vi "pwm事件.vi"(8 "error in (no error)":errorcluster caption="错误输入（无错误）", 9 "事件数据":cluster{"frequency":dbl, "duty cycle":dbl}, 10 "枚举":T1) -> (0 "error out":errorcluster, 3 "user event":refnum<user-event>)   [LabVIEW 2012]
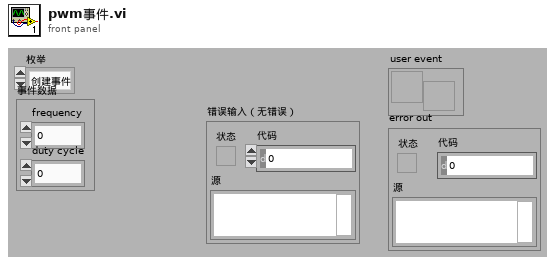
[diagram p1: front panel]
types:
  T1 = typedef "控件 2.ctl" = enum16{"创建事件", "产生事件", "销毁事件"}
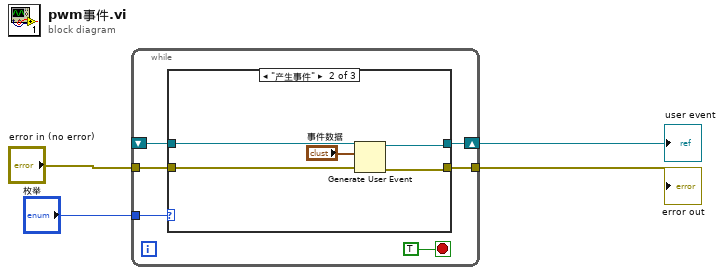
[diagram p0: block diagram]
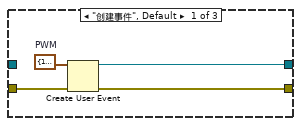
[diagram p2: hidden frame]
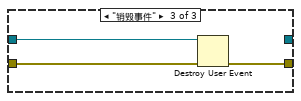
[diagram p3: hidden frame]
diagram:
  n1 = while {
    tunnel: "枚举" -> [w9]
    shift-right: [w8] -> w3
    shift-left: _ -> [w7]
    tunnel: "error in (no error)" -> [w6]
    tunnel: [w5] -> w2
    stop <- TRUE stop-if-true
    n2 = case shown="\"产生事件\"" w9 {
      tunnel: [w14 w17 _] -> w8
      tunnel: w7 -> [_ w19 w22]
      tunnel: w6 -> [w13 w16 w21]
      tunnel: [w12 w15 w20] -> w5
      frame "创建事件", Default {
        w11 = cluster{"frequency":dbl, "duty cycle":dbl} {"frequency"=100.0, "duty cycle"=0.99}  # PWM
        n3 = Create User Event(user event datatype=w11, error in=w13) -> (user event=w14:refnum<user-event>, error out=w12:errorcluster)
      }
      frame "产生事件" {
        n4 = Generate User Event(user event=w19, event data cluster="事件数据", error in=w16) -> (user event out=w17:refnum<user-event>, error out=w15:errorcluster)
      }
      frame "销毁事件" {
        n5 = Destroy User Event(user event=w22, error in=w21) -> (error out=w20:errorcluster)
      }
    }
  }
  "user event" <- w3
  "error out" <- w2
